vi "ZeroMQ_S4ICS.vi"() -> ()   [LabVIEW 2018]
uses:
  <vilib>/addons/zeromq/socket_type.ctl
  <vilib>/addons/zeromq/socket_options.ctl
  <vilib>/addons/zeromq/zeromq.lvlib
  <vilib>/addons/zeromq/zmq_socket.lvclass
  <vilib>/addons/zeromq/zmq_context.lvclass
panel:
  out "error out 2":errorcluster
  in  "stop 4":bool
  out "command 2":string
  out "error out 4":errorcluster
  out "ADDRESS SUB":string
  out "command tcpip":string
  out "error out":errorcluster
  out "command":string
  in  "stop 3":bool
  out "error out 3":errorcluster
  out "response sub":string
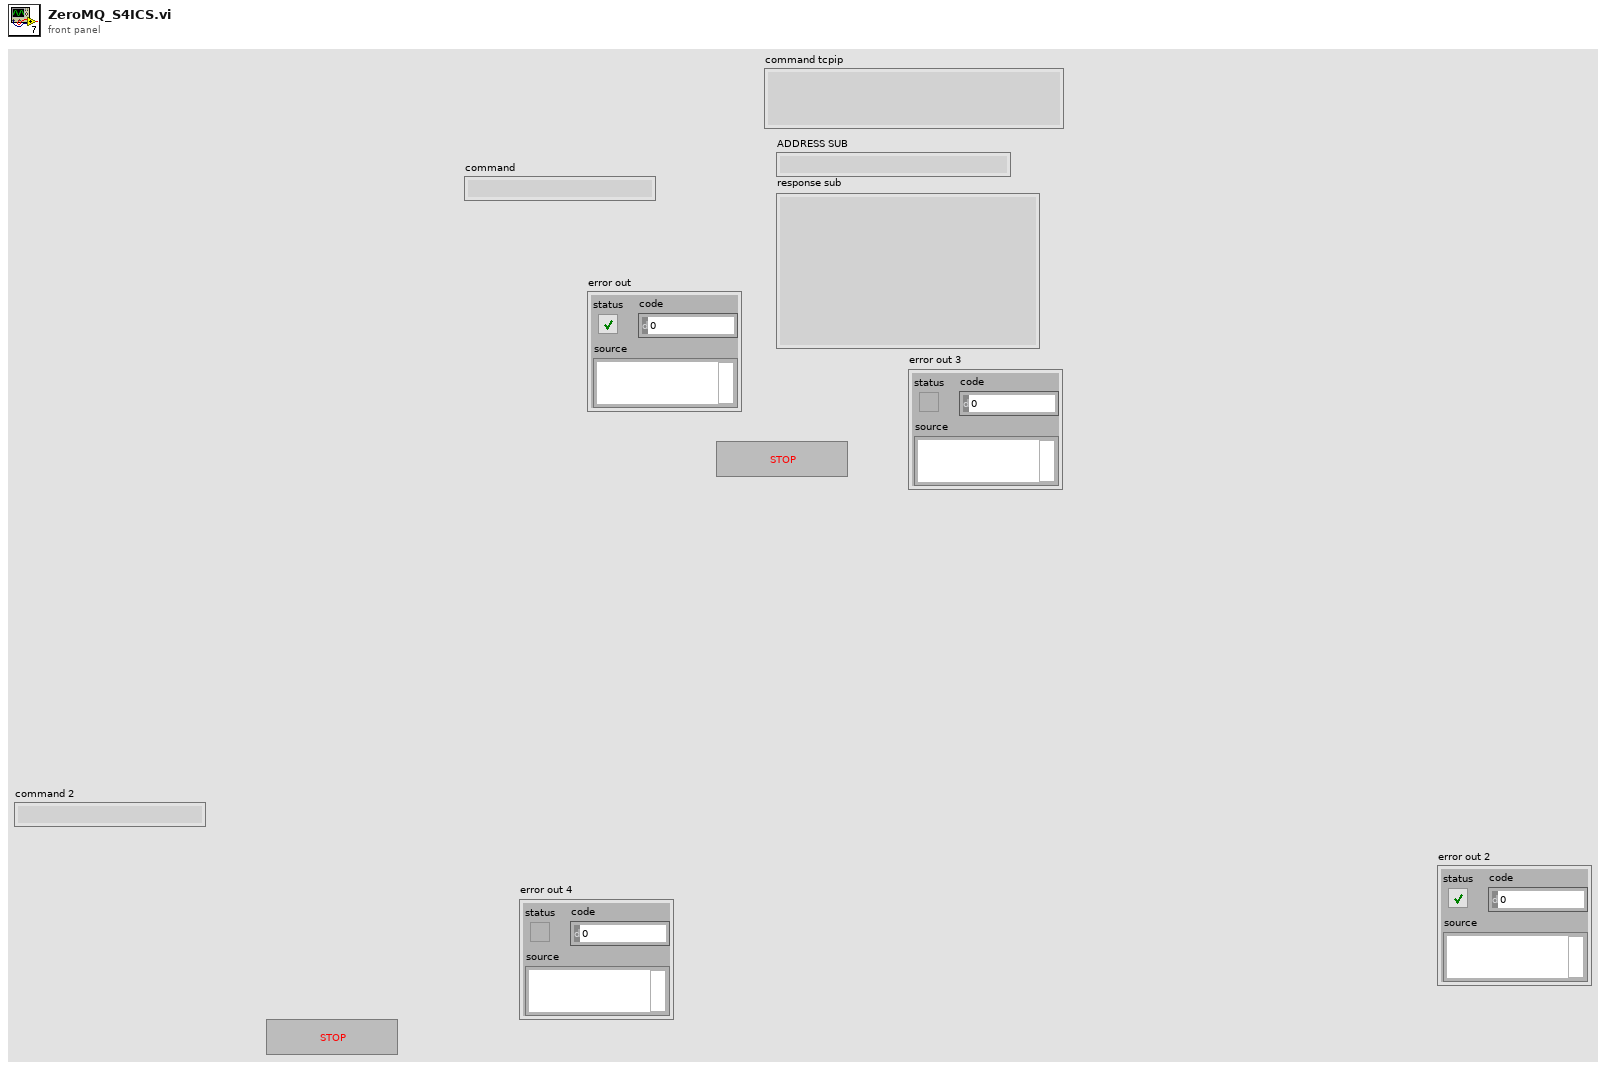
[diagram p1: front panel]
types:
  T1 = typedef "zeromq.lvlib/socket_options.ctl" = enum8{"NONE", "ZMQ_HWM", "<2>", "ZMQ_SWAP", "ZMQ_AFFINITY", "ZMQ_ROUTING_ID", "ZMQ_SUBSCRIBE", "ZMQ_UNSUBSCRIBE", "ZMQ_RATE", "ZMQ_RECOVERY_IVL", "ZMQ_MCAST_LOOP", "ZMQ_SNDBUF", "ZMQ_RCVBUF", "ZMQ_RCVMORE", "ZMQ_FD", "ZMQ_EVENTS", "ZMQ_TYPE", "ZMQ_LINGER", "ZMQ_RECONNECT_IVL", "ZMQ_BACKLOG", "ZMQ_RECOVERY_IVL_MSEC", "ZMQ_RECONNECT_IVL_MAX", "ZMQ_MAXMSGSIZE", "ZMQ_SNDHWM", "ZMQ_RCVHWM", "ZMQ_MULTICAST_HOPS", "<26>", "ZMQ_RCVTIMEO", "ZMQ_SNDTIMEO", "<29>", "<30>", "ZMQ_IPV4ONLY", "ZMQ_LAST_ENDPOINT", "ZMQ_ROUTER_MANDATORY", "ZMQ_TCP_KEEPALIVE", "ZMQ_TCP_KEEPALIVE_CNT", "ZMQ_TCP_KEEPALIVE_IDLE", "ZMQ_TCP_KEEPALIVE_INTVL", "ZMQ_TCP_ACCEPT_FILTER", "ZMQ_IMMEDIATE", "ZMQ_XPUB_VERBOSE", "ZMQ_ROUTER_RAW", "ZMQ_IPV6", "ZMQ_MECHANISM", "ZMQ_PLAIN_SERVER", "ZMQ_PLAIN_USERNAME", "ZMQ_PLAIN_PASSWORD", "ZMQ_CURVE_SERVER", "ZMQ_CURVE_PUBLICKEY", "ZMQ_CURVE_SECRETKEY", "ZMQ_CURVE_SERVERKEY", "ZMQ_PROBE_ROUTER", "ZMQ_REQ_CORRELATE", "ZMQ_REQ_RELAXED", "ZMQ_CONFLATE", "ZMQ_ZAP_DOMAIN", "ZMQ_ROUTER_HANDOVER", "ZMQ_TOS", "ZMQ_IPC_FILTER_PID", "ZMQ_IPC_FILTER_UID", "ZMQ_IPC_FILTER_GID", "ZMQ_CONNECT_ROUTING_ID", "ZMQ_GSSAPI_SERVER", "ZMQ_GSSAPI_PRINCIPAL", "ZMQ_GSSAPI_SERVICE_PRINCIPAL", "ZMQ_GSSAPI_PLAINTEXT", "ZMQ_HANDSHAKE_IVL", "<67>", "ZMQ_SOCKS_PROXY", "ZMQ_XPUB_NODROP", "ZMQ_BLOCKY", "ZMQ_XPUB_MANUAL", "ZMQ_XPUB_WELCOME_MSG", "ZMQ_STREAM_NOTIFY", "ZMQ_INVERT_MATCHING", "ZMQ_HEARTBEAT_IVL", "ZMQ_HEARTBEAT_TTL", "ZMQ_HEARTBEAT_TIMEOUT", "ZMQ_XPUB_VERBOSER", "ZMQ_CONNECT_TIMEOUT", "ZMQ_TCP_MAXRT", "ZMQ_THREAD_SAFE", "<82>", "<83>", "ZMQ_MULTICAST_MAXTPDU", "ZMQ_VMCI_BUFFER_SIZE", "ZMQ_VMCI_BUFFER_MIN_SIZE", "ZMQ_VMCI_BUFFER_MAX_SIZE", "ZMQ_VMCI_CONNECT_TIMEOUT", "ZMQ_USE_FD", "ZMQ_GSSAPI_PRINCIPAL_NAMETYPE", "ZMQ_GSSAPI_SERVICE_PRINCIPAL_NAMETYPE", "ZMQ_BINDTODEVICE", "ZMQ_ZAP_ENFORCE_DOMAIN", "ZMQ_LOOPBACK_FASTPATH", "ZMQ_METADATA", "ZMQ_MULTICAST_LOOP", "ZMQ_ROUTER_NOTIFY"}
  T2 = typedef "zeromq.lvlib/socket_type.ctl" = enum8{"ZMQ_PAIR", "ZMQ_PUB", "ZMQ_SUB", "ZMQ_REQ", "ZMQ_REP", "ZMQ_DEALER", "ZMQ_ROUTER", "ZMQ_PULL", "ZMQ_PUSH", "ZMQ_XPUB", "ZMQ_XSUB", "ZMQ_STREAM", "ZMQ_SERVER", "ZMQ_CLIENT", "ZMQ_RADIO", "ZMQ_DISH", "ZMQ_GATHER", "ZMQ_SCATTER", "ZMQ_DGRAM"}
  T3 = cluster{"ID":u32, "Address":string, "Service Name 1":string, "Service Name 2":string, "queue TX":refnum<queue>, "queue RX":refnum<queue>, "Port 1":u32, "Port 2":u32}
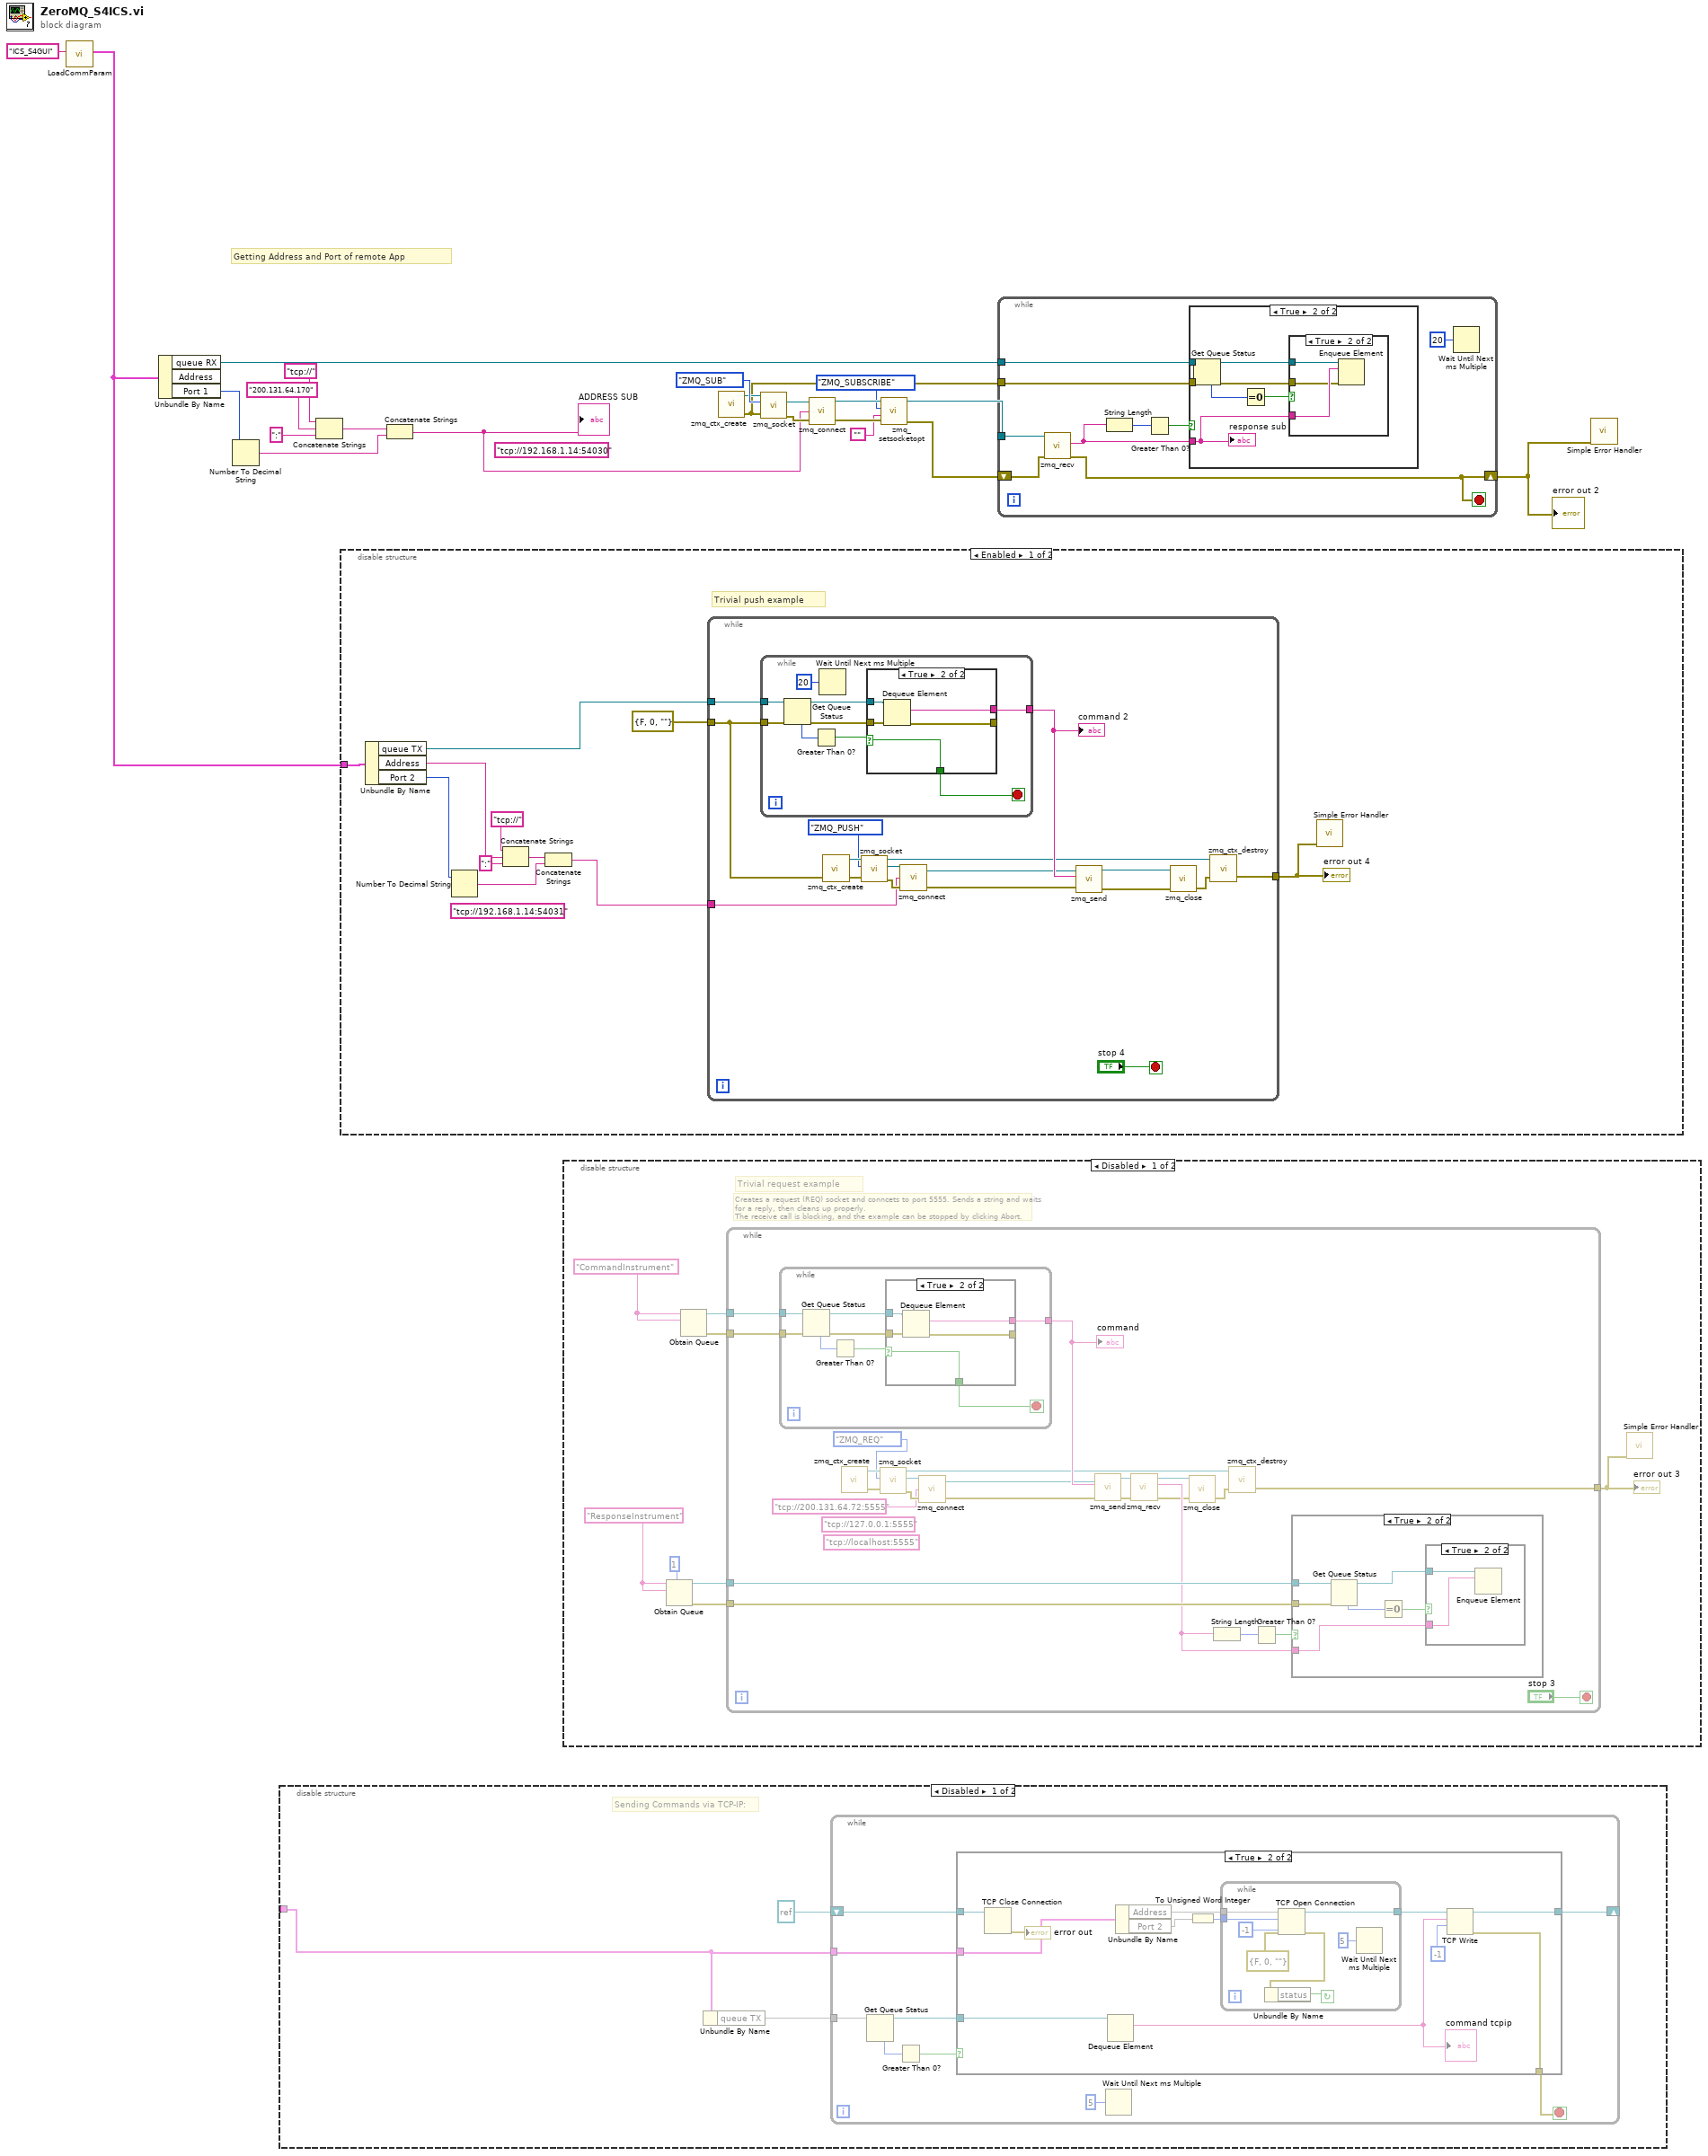
[diagram p0: block diagram]
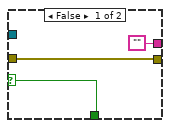
[diagram p2: hidden frame]
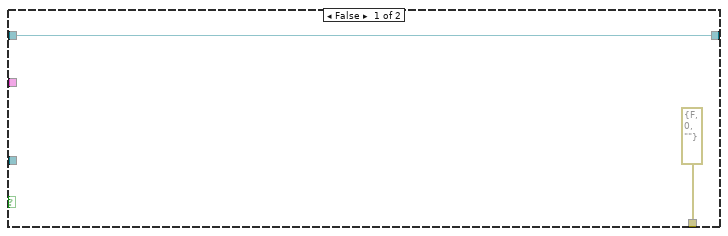
[diagram p4: hidden frame]
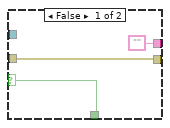
[diagram p10: hidden frame]
diagram:
  (unwired) "tcp://192.168.1.14:54030" ("endpoint")
  # "Getting Address and Port of remote App"
  n1 = call "LoadCommParam.vi"("section name"="ICS_S4GUI") -> ("output cluster"=w2:T3)  [unwired: 10 in]
  n2 = Unbundle By Name(w2) -> ("queue RX"=w9:refnum<queue>, "Port 1"=w8:u32)  [unwired: 1 out]
  n3 = Number To Decimal String(number=w8) -> (decimal integer string=w7:string)  [unwired: 1 in]
  n4 = disable-structure shown="Disabled" {
    disable-tunnel: _ -> [w23 _]
    frame Disabled {
      # "Sending Commands via TCP-IP:"
      n5 = Unbundle By Name(w23) -> ("queue TX"=w25)
      n6 = while {
        tunnel: w25 -> [w34]
        tunnel: w23 -> [w29]
        shift-right: [w27] -> _
        shift-left: refnum<k5> refnum ("connection ID") -> [w26]
        stop <- w28 stop-if-true
        n7 = Get Queue Status(queue=w34) -> (queue out=w31:refnum<queue>, # elements in queue=w33:i32)  [unwired: 2 in, 6 out]
        n8 = Greater Than 0?(x=w33) -> (x > 0?=w32:bool)
        n9 = case shown="True" w32 {
          tunnel: w31 -> [_ w48]
          tunnel: w29 -> [_ w46]
          tunnel: [errorcluster {"status"=FALSE, "code"=0, "source"=""} ("error out") w40] -> w28
          tunnel: [w35 w39] -> w27
          tunnel: w26 -> [w35 w37]
          frame False {
          }
          frame True {
            n10 = TCP Close Connection(connection ID=w37) -> (error out=→"error out":errorcluster)  [unwired: 2 in, 1 out]
            n11 = Dequeue Element(queue=w48) -> (element=w47:string)  [unwired: 2 in, 3 out]
            "command tcpip" <- w47
            n12 = Unbundle By Name(w46) -> ("Address"=w42, "Port 2"=w41)
            n13 = To Unsigned Word Integer(number=w41) -> (unsigned 16bit integer=w43:u16)
            n14 = while {
              tunnel: [w56] -> w45
              tunnel: w43 -> [w55]
              tunnel: w42 -> [w54]
              stop <- w50 continue-if-true
              n15 = TCP Open Connection(address=w54, remote port or service name=w55, timeout ms (60000)=-1, error in (no error)=errorcluster {"status"=FALSE, "code"=0, "source"=""}) -> (connection ID=w56:refnum<k5>, error out=w51:errorcluster)  [unwired: 1 in]
              n16 = Unbundle By Name(w51) -> ("status"=w50:bool)
              n17 = Wait Until Next ms Multiple(millisecond multiple=u32 5) -> ()  [unwired: 1 out]
            }
            n18 = TCP Write(connection ID=w45, data in=w47, 9:-1 ("timeout ms (25000)")) -> (connection ID out=w39:refnum<k5>, error out=w40:errorcluster)  [unwired: 1 in, 1 out]
          }
        }
        n19 = Wait Until Next ms Multiple(millisecond multiple=u32 5) -> ()  [unwired: 1 out]
      }
    }
    frame Enabled {
    }
  }
  n20 = Concatenate Strings("tcp://" ("string"), "200.131.64.170" ("string"), ":" ("string")) -> (w6:string)
  n21 = disable-structure shown="Enabled" {
    disable-tunnel: w2 -> [w57 _]
    frame Enabled {
      (unwired) "tcp://192.168.1.14:54031" ("endpoint")
      # "Trivial push example"
      n22 = Unbundle By Name(w57) -> ("queue TX"=w59:refnum<queue>, "Address"=w61:string, "Port 2"=w60:u32)
      n23 = Number To Decimal String(number=w60) -> (decimal integer string=w65:string)  [unwired: 1 in]
      n24 = Concatenate Strings("tcp://" ("string"), w61, ":" ("string")) -> (w64:string)
      n25 = Concatenate Strings(w64, w65) -> (w58:string)
      n26 = while {
        tunnel: w59 -> [w84]
        tunnel: errorcluster {"status"=FALSE, "code"=0, "source"=""} ("error out") -> [w68]
        tunnel: [w73] -> w67
        tunnel: w58 -> [w69]
        stop <- "stop 4" stop-if-true
        n27 = while {
          tunnel: w84 -> [w92]
          tunnel: w68 -> [w91]
          tunnel: [w87] -> w83
          stop <- w86 stop-if-true
          n28 = Get Queue Status(queue=w92, error in (no error)=w91) -> (queue out=w88:refnum<queue>, error out=w89:errorcluster, # elements in queue=w93:i32)  [unwired: 1 in, 5 out]
          n29 = Greater Than 0?(x=w93) -> (x > 0?=w90:bool)
          n30 = Wait Until Next ms Multiple(millisecond multiple=u32 20) -> ()  [unwired: 1 out]
          n31 = case shown="True" w90 {
            selector: w90 -> [w94 w97]
            tunnel: w89 -> [w96 w101]
            tunnel: w88 -> [_ w100]
            tunnel: [w96 w99] -> _
            tunnel: ["" w98] -> w87
            tunnel: [w94 w97] -> w86
            frame False {
            }
            frame True {
              n32 = Dequeue Element(queue=w100, error in (no error)=w101) -> (element=w98:string, error out=w99:errorcluster)  [unwired: 1 in, 2 out]
            }
          }
        }
        "command 2" <- w83
        n33 = call <vilib>:"zmq_ctx_create.vi"("error in"=w68) -> ("error out"=w78:errorcluster, "context out"=w81:refnum<class "zmq_context.lvclass">)  [unwired: 3 in]
        n34 = call <vilib>:"zmq_socket.vi"("error in"=w78, "socket type"=socket_type."ZMQ_PUSH", "context in"=w81) -> ("error out"=w80:errorcluster, "socket out"=w79:refnum<class "zmq_socket.lvclass">, "context out"=w72:refnum<class "zmq_context.lvclass">)  [unwired: 2 in]
        n35 = call <vilib>:"zmq_connect.vi"("error in"=w80, "endpoint"=w69, "socket in"=w79) -> ("error out"=w75:errorcluster, "socket out"=w76:refnum<class "zmq_socket.lvclass">)  [unwired: 1 in]
        n36 = call <vilib>:"zmq_send.vi"("error in"=w75, "data"=w83, "socket in"=w76) -> ("error out"=w70:errorcluster, "socket out"=w71:refnum<class "zmq_socket.lvclass">)  [unwired: 4 in]
        n37 = call <vilib>:"zmq_close.vi"("error in"=w70, "socket"=w71) -> ("error out"=w74:errorcluster)  [unwired: 3 in]
        n38 = call <vilib>:"zmq_ctx_destroy.vi"("error in"=w74, "context in"=w72) -> ("error out"=w73:errorcluster)  [unwired: 3 in]
      }
      "error out 4" <- w67
      n39 = call <vilib>:"Simple Error Handler.vi"("error in (no error)"=w67) -> ()  [unwired: 4 in, 5 out]
    }
    frame Disabled {
    }
  }
  n40 = Concatenate Strings(w6, w7) -> (w12:string)
  "ADDRESS SUB" <- w12
  n41 = disable-structure shown="Disabled" {
    frame Disabled {
      w102 = "ResponseInstrument"
      w103 = "CommandInstrument"
      # "Creates a request (REQ) socket and conncets to port 5555. Sends a string and waits for a reply, then cleans up properly.\nThe receive call is blocking, and the example can be stopped by clicking Abort."
      # "Trivial request example"
      n42 = Obtain Queue(max queue size (-1, unlimited)=1, name (unnamed)=w102, element data type=w102) -> (queue out=w106:refnum<queue>, error out=w105:errorcluster)  [unwired: 2 in, 1 out]
      n43 = Obtain Queue(name (unnamed)=w103, element data type=w103) -> (queue out=w108:refnum<queue>, error out=w107:errorcluster)  [unwired: 3 in, 1 out]
      n44 = while {
        tunnel: w108 -> [w131]
        tunnel: w107 -> [w130]
        tunnel: w106 -> [w128]
        tunnel: w105 -> [w127]
        tunnel: [w114] -> w104
        stop <- "stop 3" stop-if-true
        (unwired) "tcp://127.0.0.1:5555" ("endpoint")
        (unwired) "tcp://localhost:5555" ("endpoint")
        n45 = while {
          tunnel: w131 -> [w148]
          tunnel: w130 -> [w147]
          tunnel: [w143] -> w129
          stop <- w142 stop-if-true
          n46 = Get Queue Status(queue=w148, error in (no error)=w147) -> (queue out=w144:refnum<queue>, error out=w145:errorcluster, # elements in queue=w149:i32)  [unwired: 1 in, 5 out]
          n47 = Greater Than 0?(x=w149) -> (x > 0?=w146:bool)
          n48 = case shown="True" w146 {
            selector: w146 -> [w150 w153]
            tunnel: w145 -> [w152 w157]
            tunnel: w144 -> [_ w156]
            tunnel: [w152 w155] -> _
            tunnel: ["" w154] -> w143
            tunnel: [w150 w153] -> w142
            frame False {
            }
            frame True {
              n49 = Dequeue Element(queue=w156, error in (no error)=w157) -> (element=w154:string, error out=w155:errorcluster)  [unwired: 1 in, 2 out]
            }
          }
        }
        "command" <- w129
        n50 = call <vilib>:"zmq_ctx_create.vi"() -> ("error out"=w119:errorcluster, "context out"=w122:refnum<class "zmq_context.lvclass">)  [unwired: 4 in]
        n51 = call <vilib>:"zmq_socket.vi"("error in"=w119, "socket type"=socket_type."ZMQ_REQ", "context in"=w122) -> ("error out"=w121:errorcluster, "socket out"=w120:refnum<class "zmq_socket.lvclass">, "context out"=w111:refnum<class "zmq_context.lvclass">)  [unwired: 2 in]
        n52 = call <vilib>:"zmq_connect.vi"("error in"=w121, "endpoint"="tcp://200.131.64.72:5555", "socket in"=w120) -> ("error out"=w116:errorcluster, "socket out"=w117:refnum<class "zmq_socket.lvclass">)  [unwired: 1 in]
        n53 = call <vilib>:"zmq_send.vi"("error in"=w116, "data"=w129, "socket in"=w117) -> ("error out"=w132:errorcluster, "socket out"=w133:refnum<class "zmq_socket.lvclass">)  [unwired: 4 in]
        n54 = call <vilib>:"zmq_recv.vi"("error in"=w132, "socket in"=w133) -> ("error out"=w113:errorcluster, "data"=w125:string, "socket out"=w112:refnum<class "zmq_socket.lvclass">)  [unwired: 3 in, 2 out]
        n55 = call <vilib>:"zmq_close.vi"("error in"=w113, "socket"=w112) -> ("error out"=w115:errorcluster)  [unwired: 3 in]
        n56 = String Length(string=w125) -> (length=w126:i32)
        n57 = call <vilib>:"zmq_ctx_destroy.vi"("error in"=w115, "context in"=w111) -> ("error out"=w114:errorcluster)  [unwired: 3 in]
        n58 = Greater Than 0?(x=w126) -> (x > 0?=w124:bool)
        n59 = case shown="True" w124 {
          tunnel: w128 -> [_ w138]
          tunnel: w125 -> [_ w135]
          tunnel: w127 -> [_ w134]
          frame False {
          }
          frame True {
            n60 = Get Queue Status(queue=w138, error in (no error)=w134) -> (queue out=w136:refnum<queue>, # elements in queue=w139:i32)  [unwired: 1 in, 6 out]
            n61 = Equal To 0?(x=w139) -> (x = 0?=w137:bool)
            n62 = case shown="True" w137 {
              tunnel: w136 -> [_ w141]
              tunnel: w135 -> [_ w140]
              frame False {
              }
              frame True {
                n63 = Enqueue Element(queue=w141, element=w140) -> ()  [unwired: 2 in, 3 out]
              }
            }
          }
        }
      }
      "error out 3" <- w104
      n64 = call <vilib>:"Simple Error Handler.vi"("error in (no error)"=w104) -> ()  [unwired: 4 in, 5 out]
    }
    frame Enabled {
    }
  }
  n65 = call <vilib>:"zmq_ctx_create.vi"() -> ("error out"=w10:errorcluster, "context out"=w13:refnum<class "zmq_context.lvclass">)  [unwired: 4 in]
  n66 = call <vilib>:"zmq_socket.vi"("error in"=w10, "socket type"=socket_type."ZMQ_SUB", "context in"=w13) -> ("error out"=w21:errorcluster, "socket out"=w14:refnum<class "zmq_socket.lvclass">)  [unwired: 2 in, 1 out]
  n67 = call <vilib>:"zmq_connect.vi"("error in"=w21, "endpoint"=w12, "socket in"=w14) -> ("error out"=w19:errorcluster, "socket out"=w20:refnum<class "zmq_socket.lvclass">)  [unwired: 1 in]
  n68 = call <vilib>:"zmq_setsocketopt.vi"("error in"=w19, "value"="", "option"=socket_options."ZMQ_SUBSCRIBE", "socket in"=w20) -> ("error out"=w18:errorcluster, "socket out"=w17:refnum<class "zmq_socket.lvclass">)  [unwired: 2 in]
  n69 = while {
    tunnel: w17 -> [w159]
    tunnel: w9 -> [w162]
    shift-right: [w165] -> w1
    shift-left: w18 -> [w166]
    tunnel: w10 -> [w160]
    stop <- w165 stop-if-true
    n70 = call <vilib>:"zmq_recv.vi"("error in"=w166, "socket in"=w159) -> ("error out"=w165:errorcluster, "data"=w161:string)  [unwired: 3 in, 3 out]
    n71 = String Length(string=w161) -> (length=w164:i32)
    n72 = Greater Than 0?(x=w164) -> (x > 0?=w163:bool)
    n73 = case shown="True" w163 {
      tunnel: w162 -> [_ w172]
      tunnel: w161 -> [_ w169]
      tunnel: w160 -> [_ w168]
      frame False {
      }
      frame True {
        n74 = Get Queue Status(queue=w172, error in (no error)=w168) -> (queue out=w170:refnum<queue>, error out=w167:errorcluster, # elements in queue=w173:i32)  [unwired: 1 in, 5 out]
        n75 = Equal To 0?(x=w173) -> (x = 0?=w171:bool)
        n76 = case shown="True" w171 {
          tunnel: w170 -> [_ w176]
          tunnel: w169 -> [_ w175]
          tunnel: w167 -> [_ w174]
          frame False {
          }
          frame True {
            n77 = Enqueue Element(queue=w176, element=w175, error in (no error)=w174) -> ()  [unwired: 1 in, 3 out]
          }
        }
        "response sub" <- w169
      }
    }
    n78 = Wait Until Next ms Multiple(millisecond multiple=u32 20) -> ()  [unwired: 1 out]
  }
  "error out 2" <- w1
  n79 = call <vilib>:"Simple Error Handler.vi"("error in (no error)"=w1) -> ()  [unwired: 4 in, 5 out]
